vi "Wait.Gui.vi"() -> ()   [LabVIEW 2016]
uses:
  Wait.Gui.Action.ctl
panel:
  out "_loop":i32(ring)=4
  out "status":string
  out "Slide":i32(slide) scale=-1.1..-1.0
  out "message":string
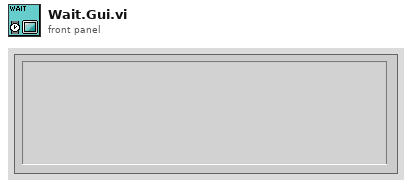
[diagram p1: front panel]
types:
  T1 = cluster{"Msg":string, "Status":string, "ProgBarSize":i32}
  T2 = enum32{"Invalid", "Standard", "Closed", "Hidden", "Minimized", "Maximized"}
  T3 = typedef "Wait.Gui.Action.ctl" = enum32{"idle", "constructor", "destructor", "--- GuiServerWait ---", "open FP", "close FP", "update msg", "update progbar"}
  T4 = typedef "LVPositionTypeDef.ctl" = cluster{"Left":i32, "Top":i32}
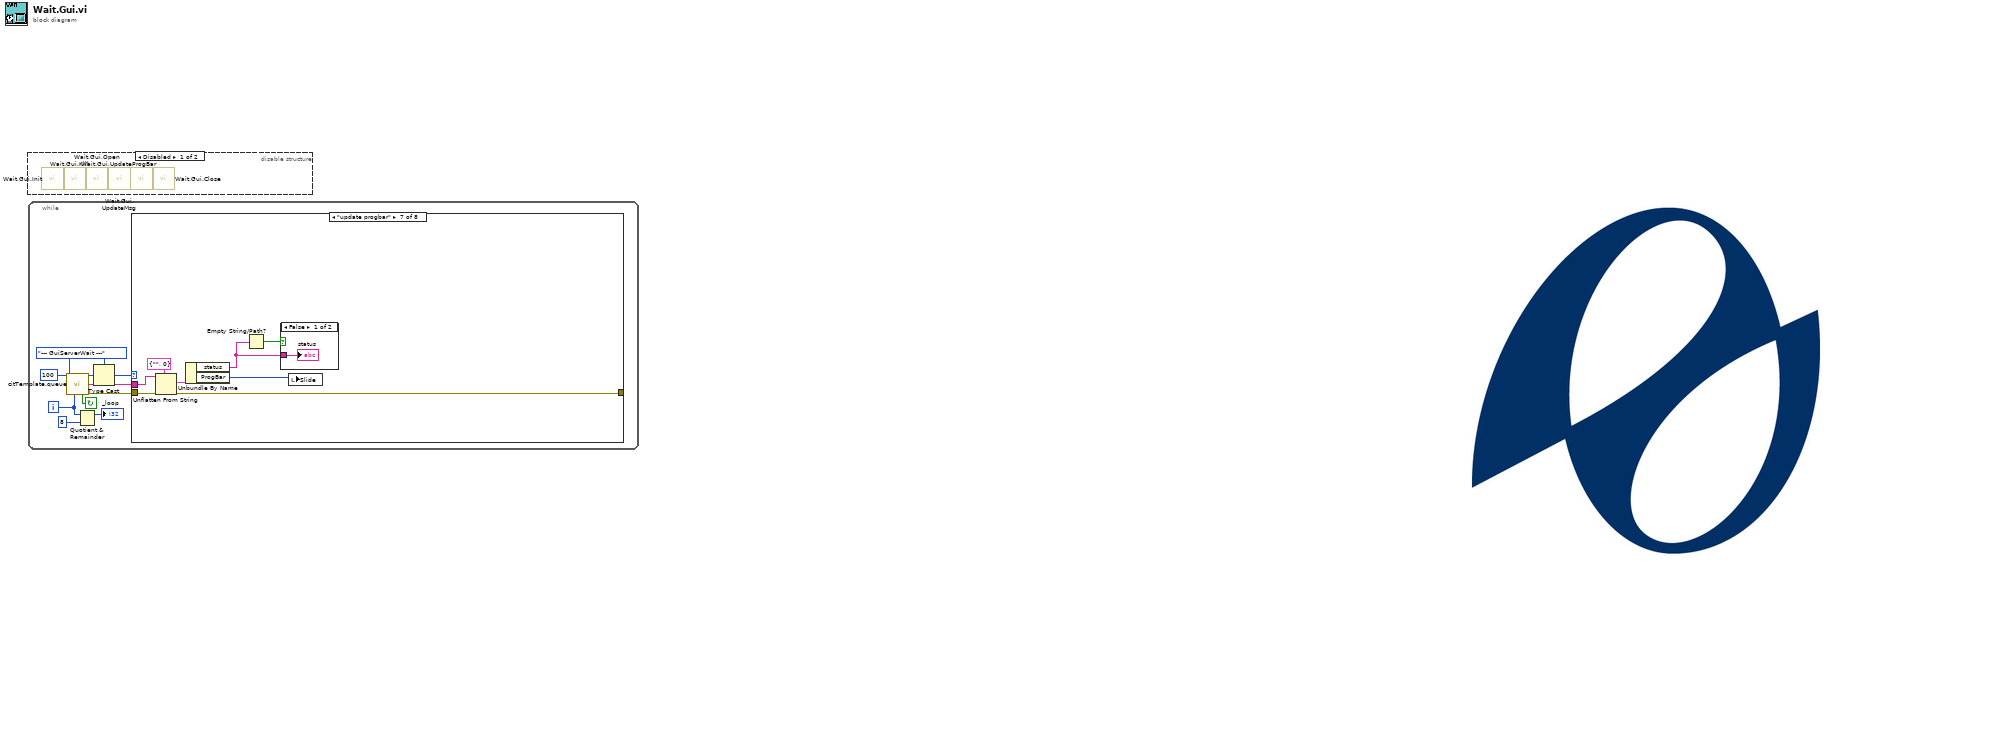
[diagram p0: block diagram]
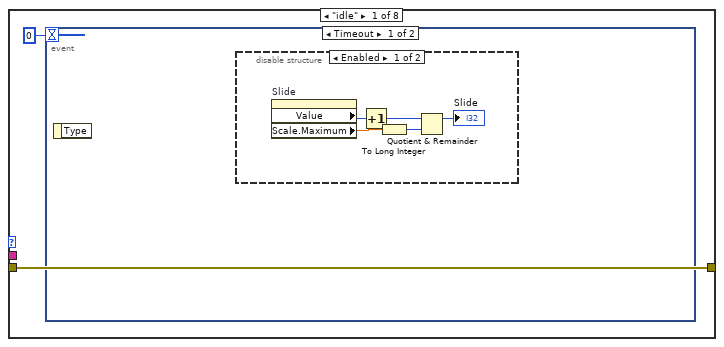
[diagram p3: hidden frame]
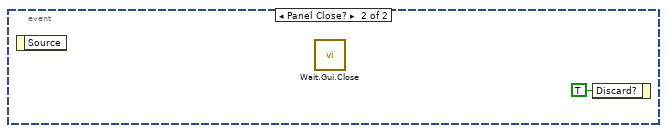
[diagram p5: hidden frame]
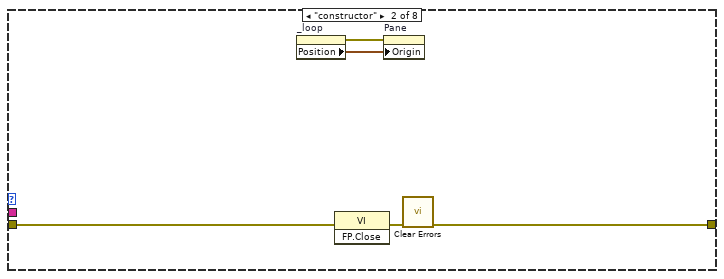
[diagram p6: hidden frame]
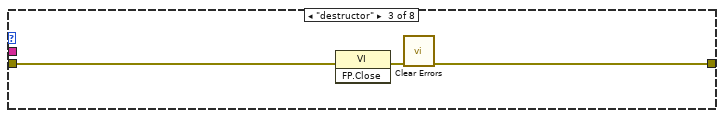
[diagram p7: hidden frame]
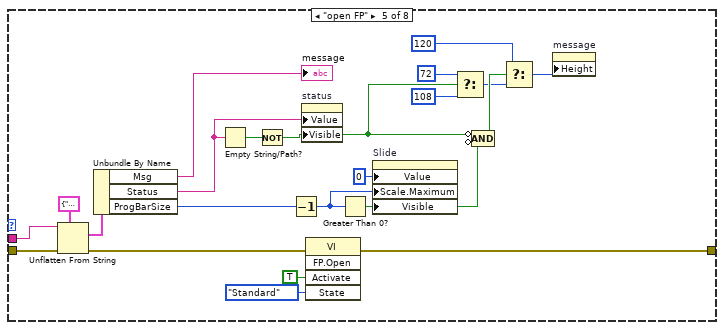
[diagram p9: hidden frame]
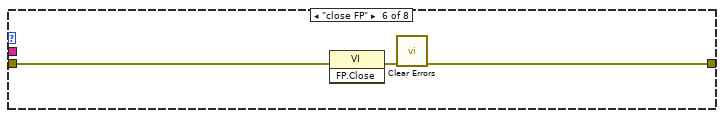
[diagram p10: hidden frame]
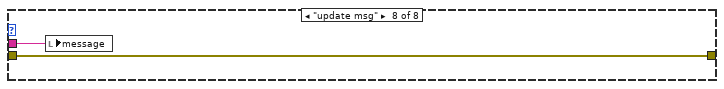
[diagram p12: hidden frame]
diagram:
  n1 = disable-structure shown="Disabled" {
    frame Disabled {
      n2 = call "Wait.Gui.Init.vi"() -> ()  [unwired: 11 in, 1 out]
      n3 = call "Wait.Gui.Kill.vi"() -> ()  [unwired: 11 in, 1 out]
      n4 = call "Wait.Gui.Open.vi"() -> ()  [unwired: 11 in, 1 out]
      n5 = call "Wait.Gui.UpdateMsg.vi"() -> ()  [unwired: 11 in, 1 out]
      n6 = call "Wait.Gui.UpdateProgBar.vi"() -> ()  [unwired: 11 in, 1 out]
      n7 = call "Wait.Gui.Close.vi"() -> ()  [unwired: 11 in, 1 out]
    }
    frame Enabled {
    }
  }
  n8 = while {
    i -> [w2]
    stop <- w4 continue-if-true
    w5 = Wait.Gui.Action."--- GuiServerWait ---" ("Action")
    n9 = call "citTemplate.queue.vi"("ms timeout (250 ms)"=100, "event enum"=w5, "iteration (-1)"=w2) -> ("event out"=w9:u32, "(flatten) data out"=w6:string, "continue"=w4:bool, "error out"=w7:errorcluster)  [unwired: 2 in, 7 out]
    n10 = Quotient & Remainder(x=w2, y=8) -> (x-y*floor(x/y)=→"_loop":i32)  [unwired: 1 out]
    n11 = Type Cast(type=w5, x=w9) -> (*(type *) &x=w8:T3)
    n12 = case shown="\"update progbar\"" w8 {
      tunnel: w7 -> [w11 w21 w26 w27 w47 w52 w60 w62]
      tunnel: w6 -> [_ _ _ _ w44 _ w59 w63]
      tunnel: [w11 w19 w24 w27 w46 w50 w58 w62] -> _
      frame "idle" {
        n13 = event shown="[0] Timeout" {
          selector: _ -> [_ _]
          dyn-events: _ -> [_ _]
          timeout: 0 -> [_ _]
          event Timeout {
            n14 = event-data() -> ()  [unwired: 1 in, 1 out]
            n15 = disable-structure shown="Enabled" {
              frame Enabled {
                n16 = property on="Slide" class="Slide (strict)"() -> ("Value"=w15:i32, "Scale.Maximum"=w16:dbl)  [unwired: 2 in, 2 out]
                n17 = Increment(x=w15) -> (x+1=w14:i32)
                n18 = To Long Integer(number=w16) -> (32bit integer=w17:i32)
                n19 = Quotient & Remainder(x=w14, y=w17) -> (x-y*floor(x/y)=→"Slide":i32)  [unwired: 1 out]
              }
              frame Disabled {
              }
            }
          }
          event Panel Close? {
            n20 = event-data() -> ()  [unwired: 1 in, 1 out]
            n21 = call "Wait.Gui.Close.vi"() -> ()  [unwired: 11 in, 1 out]
            n22 = event-data("Discard?"=TRUE) -> ()  [unwired: 1 in, 1 out]
          }
        }
      }
      frame "constructor" {
        n23 = property on="_loop" class="Ring (strict)"() -> (error out=w22:errorcluster, "Position"=w23:T4)  [unwired: 2 in, 1 out]
        n24 = invoke class="VI" method="FP.Close"(error in=w21) -> (error out=w20:errorcluster)  [unwired: 2 in, 2 out]
        n25 = property on="Pane" class="Pane"(error in=w22, "Origin"=w23) -> ()  [unwired: 1 in, 2 out]
        n26 = call <vilib>:"Clear Errors.vi"("error in (no error)"=w20) -> ("error out"=w19:errorcluster)  [unwired: 5 in, 1 out]
      }
      frame "destructor" {
        n27 = invoke class="VI" method="FP.Close"(error in=w26) -> (error out=w25:errorcluster)  [unwired: 2 in, 2 out]
        n28 = call <vilib>:"Clear Errors.vi"("error in (no error)"=w25) -> ("error out"=w24:errorcluster)  [unwired: 5 in, 1 out]
      }
      frame "--- GuiServerWait ---" {
      }
      frame "open FP" {
        n29 = Unflatten From String(type=T1 {"Msg"="", "Status"="", "ProgBarSize"=0} ("output cluster"), binary string=w44, error in (no error)=w47) -> (value=w42:T1, error out=w45:errorcluster)  [unwired: 2 in, 1 out]
        n30 = Unbundle By Name(w42) -> ("Msg"=→"message":string, "Status"=w37:string, "ProgBarSize"=w41:i32)
        n31 = Empty String/Path?(string/path=w37) -> (empty?=w36:bool)
        n32 = Not(x=w36) -> (.not. x?=w33:bool)
        n33 = Decrement(x=w41) -> (x-1=w40:i32)
        n34 = property on="status" class="Str"("Value"=w37, "Visible"=w33) -> ()  [unwired: 2 in, 2 out]
        n35 = invoke class="VI" method="FP.Open"(error in=w45, "Activate"=TRUE ("Activate?"), "State"=T2."Standard") -> (error out=w46:errorcluster)  [unwired: 2 in, 4 out]
        n36 = Greater Than 0?(x=w40) -> (x > 0?=w32:bool)
        n37 = property on="Slide" class="Slide (strict)"("Value"=0 ("Slide"), "Scale.Maximum"=w40, "Visible"=w32) -> ()  [unwired: 2 in, 2 out]
        n38 = Select(t=u32 72 ("Size:Height"), s=w33, f=u32 108 ("Size:Height")) -> (s? t:f=w29:u32)
        n39 = Compound Arithmetic op=AND(invert w33, invert w32) -> (w30:bool)
        n40 = Select(t=u32 120 ("Size:Height"), s=w30, f=w29) -> (s? t:f=w31:u32)
        n41 = property on="message" class="Str"("Height"=w31) -> ()  [unwired: 2 in, 2 out]
      }
      frame "close FP" {
        n42 = invoke class="VI" method="FP.Close"(error in=w52) -> (error out=w51:errorcluster)  [unwired: 2 in, 2 out]
        n43 = call <vilib>:"Clear Errors.vi"("error in (no error)"=w51) -> ("error out"=w50:errorcluster)  [unwired: 5 in, 1 out]
      }
      frame "update progbar" {
        n44 = Unflatten From String(type=cluster{"status":string, "ProgBar":i32} {"status"="", "ProgBar"=0} ("output cluster"), binary string=w59, error in (no error)=w60) -> (value=w56:cluster{"status":string, "ProgBar":i32}, error out=w58:errorcluster)  [unwired: 2 in, 1 out]
        n45 = Unbundle By Name(w56) -> ("status"=w53:string, "ProgBar"=w55:i32)
        n46 = Empty String/Path?(string/path=w53) -> (empty?=w54:bool)
        n47 = case shown="False" w54 {
          tunnel: w53 -> [w61 _]
          frame False {
            "status" <- w61
          }
          frame True {
          }
        }
        n48 = local write "Slide"(w55) -> ()
      }
      frame "update msg" {
        n49 = local write "message"(w63) -> ()
      }
    }
  }
